vi "Point Data Updated.vi"(8 "error in":errorcluster, 9 "Data":variant, 10 "Task-Point Ident":string, 11 "Series Actor in":refnum<class "Series Actor.lvclass">) -> (0 "error out":errorcluster, 3 "Series Actor out":refnum<class "Series Actor.lvclass">)   [LabVIEW 2024, in "Series Actor.lvlib" / "Series Actor.lvclass"]
doc: "Use this VI to update Point Data for repeatedly self calling Do.VI's"
uses:
  Series Actor.lvclass
  Series Actor.lvclass/Series Actor.ctl
  Data Logger Actor/Data Logger Actor/IData Logger Actor Messages/Log Data Msg/Log Data Msg.lvclass
  <vilib>/ActorFramework/Message Enqueuer/Message Enqueuer.lvclass
  ISeries UI Actor/ISeries UI Actor Messages/Point Data Updated Msg/Point Data Updated Msg.lvclass
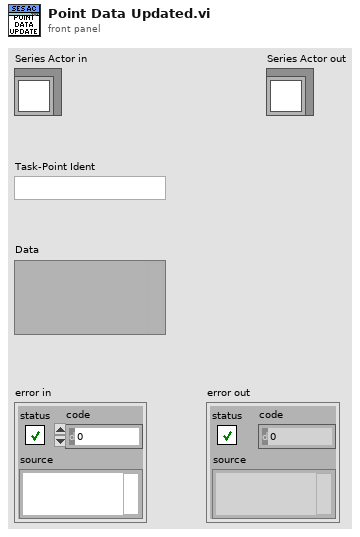
[diagram p1: front panel]
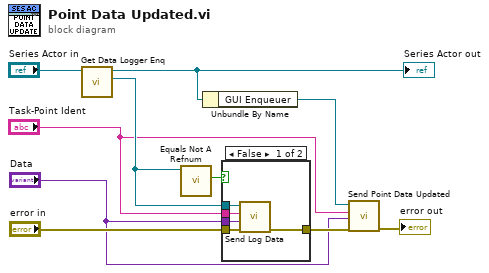
[diagram p0: block diagram]
diagram:
  n1 = call "Get Data Logger Enq.vi"("Series Actor in"="Series Actor in") -> ("Data Logger Enq"=w9:refnum<class "Message Enqueuer.lvclass">, "Series Actor out"=w1:refnum<class "Series Actor.lvclass">)  [unwired: 9 in]
  "Series Actor out" <- w1
  n2 = call <vilib>:"Equals Not A Refnum.vi"("Message Enqueuer"=w9) -> ("Not a refnum?"=w10:bool)  [unwired: 10 in]
  n3 = Unbundle By Name(w1) -> ("GUI Enqueuer"=w7:refnum<class "Message Enqueuer.lvclass">)
  n4 = case shown="False" w10 {
    tunnel: w9 -> [w15 _]
    tunnel: "Task-Point Ident" -> [w14 _]
    tunnel: "error in" -> [w12 w16]
    tunnel: [w13 w16] -> w8
    tunnel: "Data" -> [w11 _]
    frame False {
      n5 = call "Send Log Data.vi"("error in (no error)"=w12, "Data"=w11, "Ident"=w14, "Message Enqueuer"=w15) -> ("error out"=w13:errorcluster)  [unwired: 6 in, 1 out]
    }
    frame True {
    }
  }
  n6 = call "Send Point Data Updated.vi"("error in (no error)"=w8, "Data"="Data", "Task-Point Ident"="Task-Point Ident", "Message Enqueuer"=w7) -> ("error out"=→"error out":errorcluster)  [unwired: 6 in, 1 out]
